vi "compare-stg-pos_w-msg.vi"(10 "stage positions":T2, 11 "element":T1) -> (2 "no-change":bool, 3 "output message":string)   [LabVIEW 2024]
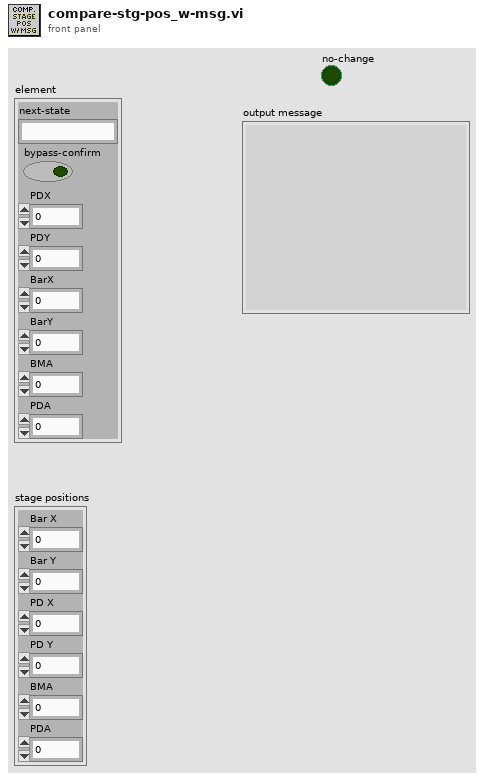
[diagram p1: front panel]
types:
  T1 = cluster{"next-state":string, "bypass-confirm":bool, "PDX":dbl, "PDY":dbl, "BarX":dbl, "BarY":dbl, "BMA":dbl, "PDA":dbl}
  T2 = cluster{"Bar X":dbl, "Bar Y":dbl, "PD X":dbl, "PD Y":dbl, "BMA":dbl, "PDA":dbl}
  T3 = cluster{"BarX":dbl, "BarY":dbl, "PDX":dbl, "PDY":dbl, "BMA":dbl, "PDA":dbl}
  T4 = cluster{bool, bool, bool, bool, "BMA":bool, "PDA":bool}
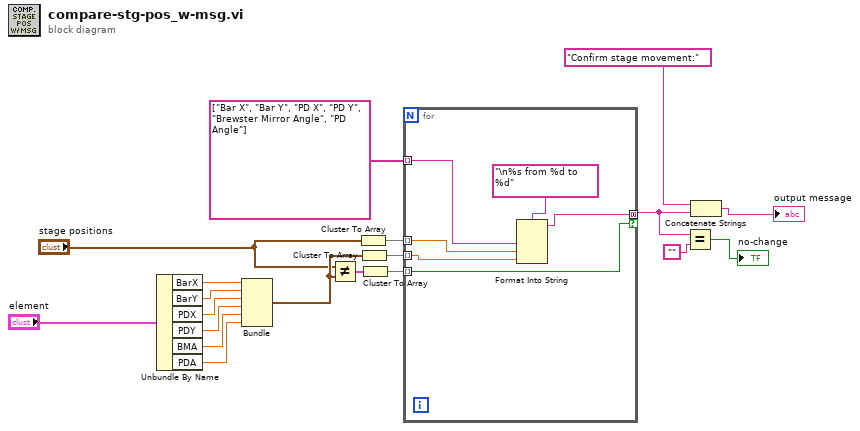
[diagram p0: block diagram]
diagram:
  n1 = Unbundle By Name("element") -> ("BarX"=w7:dbl, "BarY"=w8:dbl, "PDX"=w9:dbl, "PDY"=w10:dbl, "BMA"=w11:dbl, "PDA"=w12:dbl)
  n2 = Bundle("BarX"=w7, "BarY"=w8, "PDX"=w9, "PDY"=w10, "BMA"=w11, "PDA"=w12) -> (w18:T3)  [unwired: 1 in]
  n3 = Not Equal?(x="stage positions", y=w18) -> (x != y?=w13:T4)
  n4 = Cluster To Array(cluster="stage positions") -> (array=w17:dbl[])
  n5 = Cluster To Array(cluster=w18) -> (array=w19:dbl[])
  n6 = Cluster To Array(cluster=w13) -> (array=w14:bool[])
  n7 = for {
    tunnel: w14 -> [w25] mode=indexing
    tunnel: string[] ["Bar X", "Bar Y", "PD X", "PD Y", "Brewster Mirror Angle", "PD Angle"] -> [w23] mode=indexing
    tunnel: w17 -> [w22] mode=indexing
    tunnel: w19 -> [w21] mode=indexing
    tunnel: [w20] -> w3 mode=concatenating if=w25
    n8 = Format Into String(format string="\n%s from %d to %d" ("string"), w23, w22, w21) -> (resulting string=w20:string)  [unwired: 2 in, 1 out]
  }
  n9 = Equal?(x=w3, y="") -> (x = y?=→"no-change":bool)
  n10 = Concatenate Strings("Confirm stage movement:" ("string"), w3) -> (→"output message":string)
